vi "TurbineMultiblock.vi"(7 "Turbine Build Properties":T2 {"Energy Capacity (FE)" format="%.2f"}, 11 "Port States In":T1) -> (3 "Port States Out":T1)   [LabVIEW 2026]
uses:
  Turbine Build Properties.ctl
  Port Defs/Turbine Port States.ctl
panel:
  out "Steam (mB/t)":i64
  in  "Dumping Mode":enum16{"Idle", "Dumping Excess", "Dumping"}(ring)
  out "Steam Flow Rate (kg/s)":dbl(knob) scale=0.0..12000.0 scale format="%#_6p"
  out "Steam Inlet Rate (kg/s)":dbl(knob) scale=0.0..12000.0 scale format="%#_6p"
  out "Exhaust Pressure (bar)":dbl(knob) scale=0.0..100.0
  out "Water Flow Rate (m³/s)":dbl(knob) scale=0.0..500000.0 scale format="%#_6p"
  out "Inlet Pressure (bar)":dbl(knob) scale=0.0..100.0
  out "Energy (FE)":ext(slide) scale=-1.0..33292800000.0 scale format="%#_12f"
  out "Steam (mB)":i64(slide) max=201600000 scale=-1.0..36992000.0
  out "Water Return (mB/t)":i64
  out "Rotation":dbl format="%#_6f"
  out "Energy Production (FE/t)":ext format="%#.6p"
  out "Flow (mB/t)":i64
  # "1"
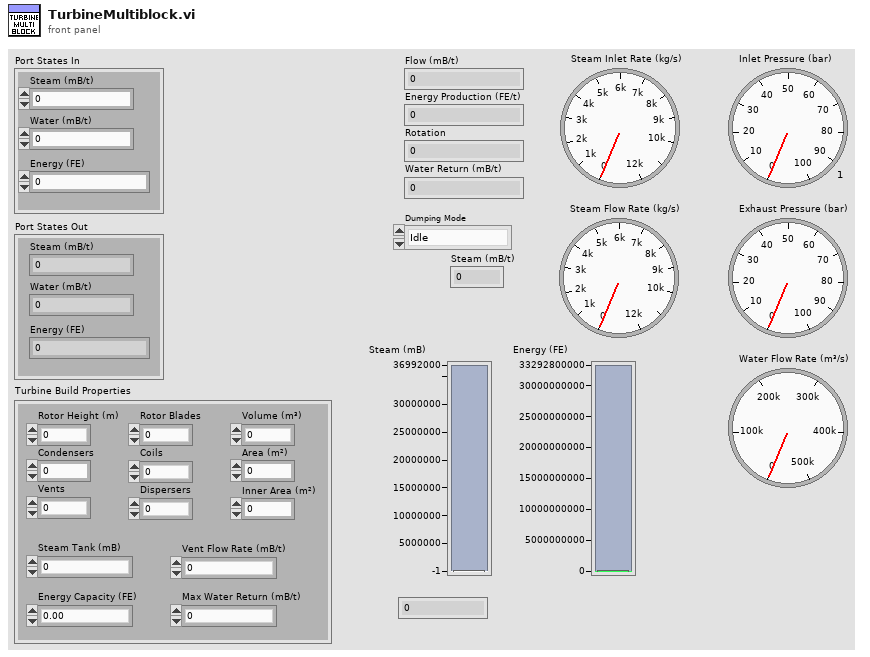
[diagram p1: front panel]
types:
  T1 = typedef "Turbine Port States.ctl" = cluster{"Steam (mB/t)":i64, "Water (mB/t)":i64, "Energy (FE)":ext}
  T2 = typedef "Turbine Build Properties.ctl" = cluster{"Volume (m³)":i32, "Rotor Height (m)":i32, "Condensers":i32, "Vents":i32, "Rotor Blades":i32, "Coils":i32, "Dispersers":i32, "Steam Tank (mB)":i64, "Energy Capacity (FE)":ext, "Vent Flow Rate (mB/t)":dbl, "Max Water Return (mB/t)":i32, "Area (m²)":i32, "Inner Area (m²)":i32}
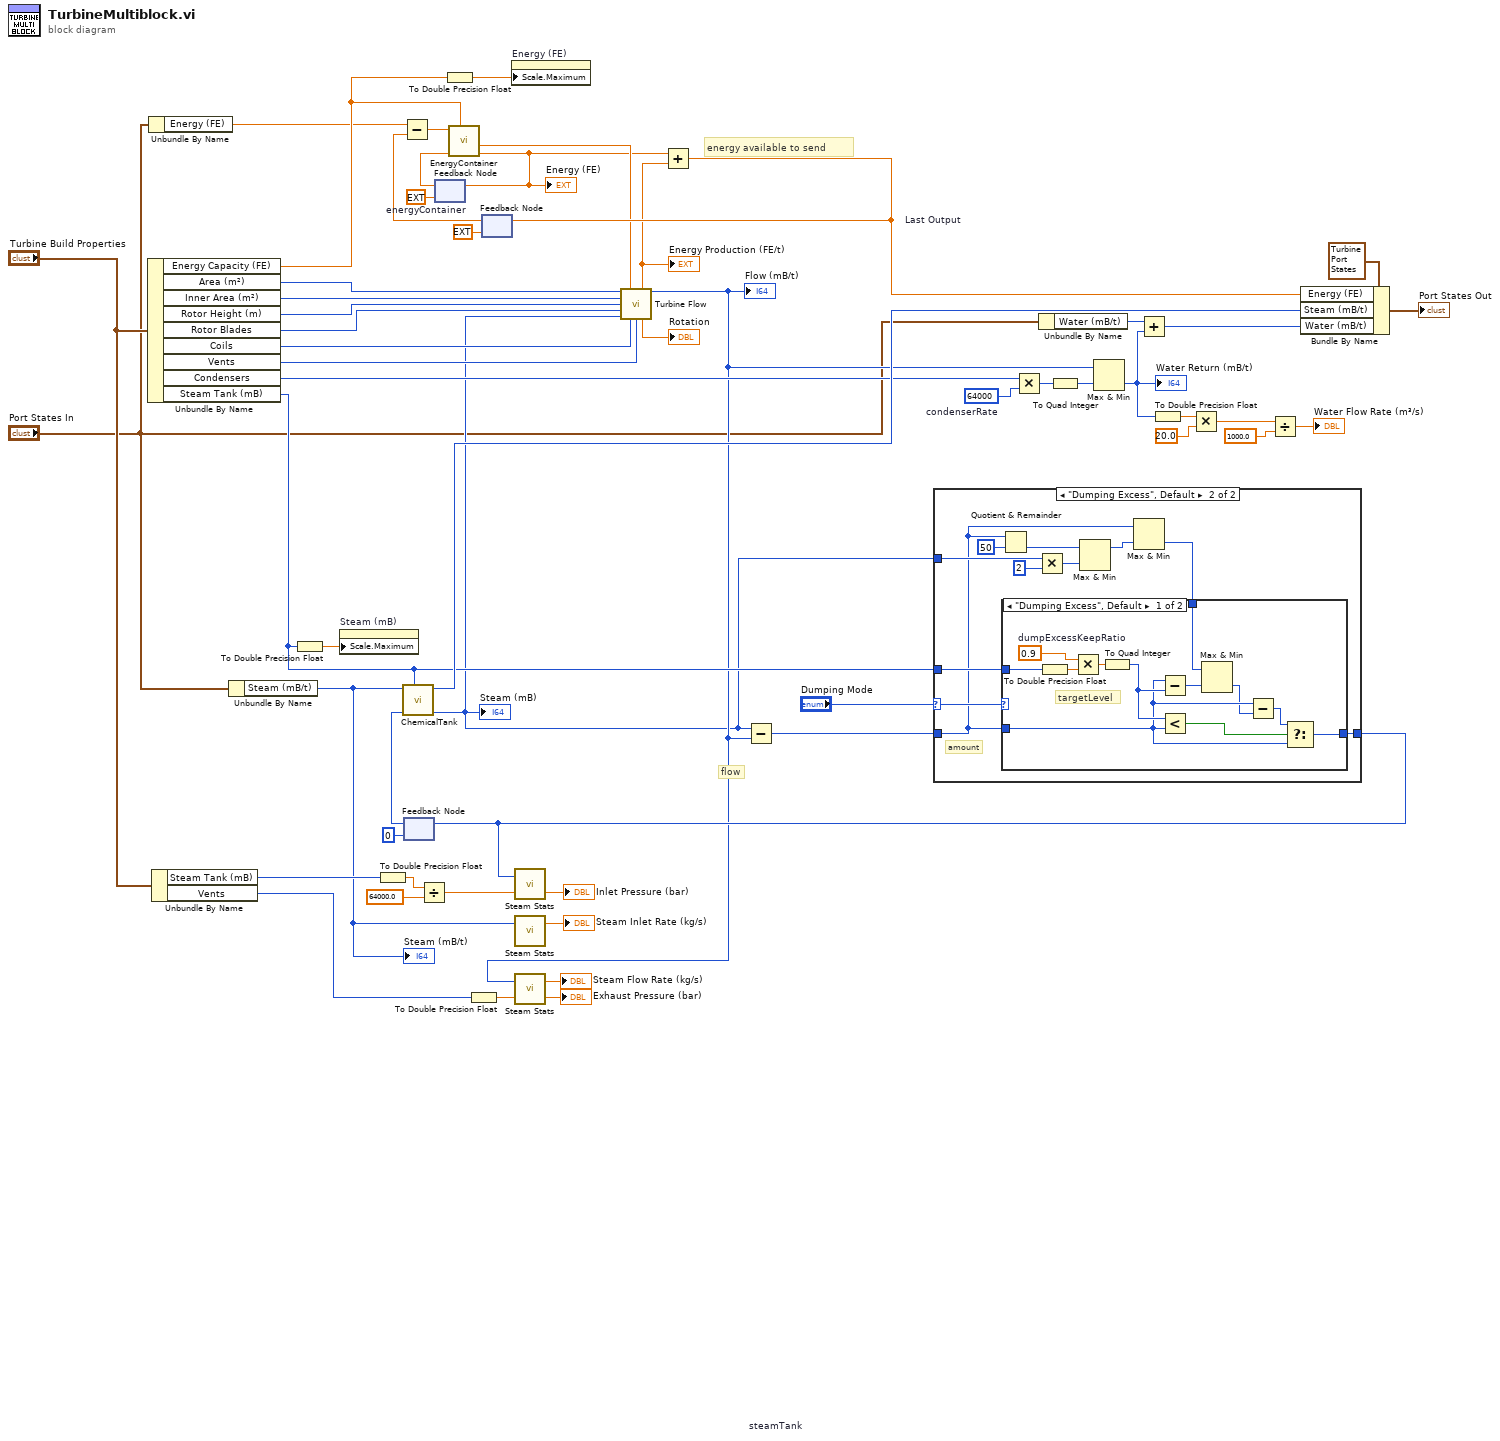
[diagram p0: block diagram]
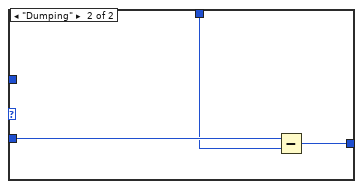
[diagram p3: hidden frame]
diagram:
  w43 = 64000  # condenserRate
  # "energy available to send"
  # "flow"
  n1 = Unbundle By Name("Turbine Build Properties") -> ("Energy Capacity (FE)"=w51:ext, "Area (m²)"=w50:i32, "Inner Area (m²)"=w49:i32, "Rotor Height (m)"=w48:i32, "Rotor Blades"=w47:i32, "Coils"=w46:i32, "Vents"=w32:i32, "Condensers"=w52:i32, "Steam Tank (mB)"=w15:i64)
  n2 = Unbundle By Name("Port States In") -> ("Energy (FE)"=w2:ext)
  n3 = Unbundle By Name("Turbine Build Properties") -> ("Steam Tank (mB)"=w21:i64, "Vents"=w22:i32)
  n4 = Unbundle By Name("Port States In") -> ("Steam (mB/t)"=w14:i64)
  "Steam (mB/t)" <- w14
  n5 = To Double Precision Float(number=w15) -> (double precision float=w29:dbl)
  n6 = property on="Steam (mB)" class="Slide (strict)"("Scale.Maximum"=w29) -> ()  [unwired: 2 in, 2 out]
  n7 = To Double Precision Float(number=w21) -> (double precision float=w26:dbl)
  n8 = feedback #1 "steamTank"(i64 0 ("Fill (mB)")) -> (w45:i64)
  n9 = call "ChemicalTank.vi"("Capacity (mB)"=w15, "Last Fill (mB)"=w45, "Transfer (mB)"=w14) -> ("Fill (mB)"=w8:i64, "Overflow (mB)"=w53:i64)  [unwired: 2 in, 2 out]
  "Steam (mB)" <- w8
  n10 = Divide(x=w26, y=64000.0) -> (x/y=w11:dbl)
  n11 = feedback #2 "energyContainer"(ext 0.0 ("Fill (FE)")) -> (w40:ext)
  n12 = To Double Precision Float(number=w51) -> (double precision float=w30:dbl)
  n13 = To Double Precision Float(number=w22) -> (double precision float=w20:dbl)
  n14 = feedback #3 "Last Output"(ext 0.0 ("Energy Production (FE)")) -> (w3:ext)
  n15 = Subtract(x=w2, y=w3) -> (x-y=w1:ext)
  n16 = call "EnergyContainer.vi"("Capacity (FE)"=w51, "Last Fill (FE)"=w40, "Transfer (FE)"=w1) -> ("Fill (FE)"=w54:ext, "Needed (FE)"=w55:ext)  [unwired: 2 in, 2 out]
  "Energy (FE)" <- w54
  n17 = feedback-in #2(w54) -> ()
  n18 = property on="Energy (FE)" class="Slide (strict)"("Scale.Maximum"=w30) -> ()  [unwired: 2 in, 2 out]
  n19 = call "Steam Stats.vi"("Flow"=w14) -> ("Flow (kg/s)"=→"Steam Inlet Rate (kg/s)":dbl)  [unwired: 1 in, 1 out]
  n20 = call "Turbine Flow.vi"("Structure Area (m²)"=w50, "Energy Needed (FE)"=w55, "Inner Area (m²)"=w49, "Rotor Height (m)"=w48, "Blades"=w47, "Stored Gas (mB/t)"=w8, "Coils"=w46, "Vents"=w32) -> ("Energy Production (FE/t)"=w4:ext, "Flow (mB/t)"=w9:i64, "Rotation"=→"Rotation":dbl)  [unwired: 1 in, 4 out]
  "Flow (mB/t)" <- w9
  "Energy Production (FE/t)" <- w4
  n21 = call "Steam Stats.vi"("Divisor"=w20, "Flow"=w9) -> ("Pressure (bar)"=→"Exhaust Pressure (bar)":dbl, "Flow (kg/s)"=→"Steam Flow Rate (kg/s)":dbl)
  n22 = Add(x=w54, y=w4) -> (x+y=w56:ext)
  n23 = feedback-in #3(w56) -> ()
  n24 = Subtract(x=w8, y=w9) -> (x-y=w17:i64)
  n25 = case shown="\"Dumping Excess\", Default" "Dumping Mode" {
    selector: "Dumping Mode" -> [_ w67]
    tunnel: w17 -> [w57 w59]
    tunnel: [w57 w66] -> w16
    tunnel: w15 -> [_ w65]
    tunnel: w8 -> [_ w68]
    frame "Idle" {
    }
    frame "Dumping Excess", Default {
      # "amount"
      n26 = Quotient & Remainder(x=w59, y=i64 50) -> (floor(x/y)=w64:i64)  [unwired: 1 out]
      n27 = Multiply(x=w68, y=i64 2) -> (x*y=w62:i64)
      n28 = Max & Min(x=w64, y=w62) -> (max(x,y)=w60:i64)  [unwired: 1 out]
      n29 = Max & Min(x=w59, y=w60) -> (min(x,y)=w58:i64)  [unwired: 1 out]
      n30 = case shown="\"Dumping Excess\", Default" w67 {
        tunnel: w59 -> [w71 w83]
        tunnel: [w75 w81] -> w66
        tunnel: w65 -> [w80 _]
        tunnel: w58 -> [w74 w82]
        frame "Dumping Excess", Default {
          w78 = 0.9  # dumpExcessKeepRatio
          # "targetLevel"
          n31 = To Double Precision Float(number=w80) -> (double precision float=w79:dbl)
          n32 = Multiply(x=w78, y=w79) -> (x*y=w77:dbl)
          n33 = To Quad Integer(1:w77) -> (0:w73:i64)
          n34 = Subtract(x=w71, y=w73) -> (x-y=w72:i64)
          n35 = Less?(x=w73, y=w71) -> (x < y?=w76:bool)
          n36 = Max & Min(x=w74, y=w72) -> (min(x,y)=w70:i64)  [unwired: 1 out]
          n37 = Subtract(x=w71, y=w70) -> (x-y=w69:i64)
          n38 = Select(t=w69, s=w76, f=w71) -> (s? t:f=w75:i64)
        }
        frame "Dumping" {
          n39 = Subtract(x=w83, y=w82) -> (x-y=w81:i64)
        }
      }
    }
  }
  n40 = feedback-in #1(w16) -> ()
  n41 = call "Steam Stats.vi"("Divisor"=w11, "Flow"=w16) -> ("Pressure (bar)"=→"Inlet Pressure (bar)":dbl)  [unwired: 1 out]
  n42 = Multiply(x=w52, y=w43) -> (x*y=w41:i32)
  n43 = Unbundle By Name("Port States In") -> ("Water (mB/t)"=w13:i64)
  n44 = To Quad Integer(1:w41) -> (0:w42:i64)
  n45 = Max & Min(x=w9, y=w42) -> (min(x,y)=w12:i64)  [unwired: 1 out]
  "Water Return (mB/t)" <- w12
  n46 = Add(x=w13, y=w12) -> (x+y=w10:i64)
  n47 = To Double Precision Float(number=w12) -> (double precision float=w19:dbl)
  n48 = Multiply(x=w19, y=20.0) -> (x*y=w36:dbl)
  n49 = Divide(x=w36, y=1000.0) -> (x/y=→"Water Flow Rate (m³/s)":dbl)
  n50 = Bundle By Name(cluster=T1 {"Steam (mB/t)"=0, "Water (mB/t)"=0, "Energy (FE)"=0.0} ("Port States In"), "Energy (FE)"=w56, "Steam (mB/t)"=w53, "Water (mB/t)"=w10) -> (→"Port States Out":T1)
